vi "niFpgaTargetMethod_MergeVI.vi"   [LabVIEW 2017]
doc: "Invokes a method on an FPGA target in the Project Explorer window. The available methods depend on the FPGA target and some FPGA targets do not support any methods."
uses:
  <vilib>/eio/EIOMethodNode/EIOMethodNode.xnode
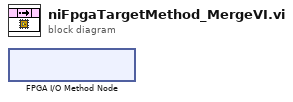
[diagram p0: block diagram]
diagram:
  n1 = xnode "FPGA I/O Method Node"() -> ()  [unwired: 1 in, 1 out]
